vi "Processing.vi"() -> ()   [LabVIEW 2016]
uses:
  Processing/results_data.ctl
  MainFGV/Settings/Advanced/AdvancedConfig.ctl
  Post_processing/GraphMean/data_mean_plot.ctl
  Post_processing/GraphMean/plot_props.ctl
  Post_processing/GraphMean/axis_props.ctl
  <vilib>/Heliosphere Research LLC/Advanced Plotting Toolkit/api_core/NewPlotScales.ctl
  <vilib>/Analysis/NI_AALPro.lvlib
  <vilib>/Heliosphere Research LLC/Advanced Plotting Toolkit/Advanced Plotting Toolkit.lvlib
panel:
  in  "stop":bool
  in  "ranges":T1(array[cluster])=[{"minFreq"=0.0, "maxFreq"=1000.0, "alpha"=20.0}] caption="Ranges de procura de picos" {"alpha" min=0.0 max=100.0 format="%#_6f %"; "maxFreq" format="%#_g Hz"; "minFreq" format="%#_g Hz"}
  in  "log":bool
  in  "alpha":dbl=0.3 caption="Alpha" format="%#_6f"
  in  "maxFreq":dbl=72.0 caption="Frequência máxima" format="%#_g Hz"
  in  "minFreq":dbl=30.0 caption="Frequência mínima" format="%#_g Hz"
  in  "lowPass":dbl=1000.0 caption="Passa baixa" format="%#_g Hz"
  in  "highPass":dbl=1.0 caption="Passa alta" format="%#_g Hz"
  in  "Filtro":T2(ring)=enum."Passa banda"
  in  "cutoff":dbl=-6.0 caption="Cutoff amplitude [dB]" format="%#_g dB"
  in  "delete":bool
  in  "ok":bool
  in  "validate":bool
  in  "tab":T3(tab)
  out "inert":waveform(dbl)[](graph) caption="Inertância"
  out "hammerSpec":waveform(dbl)(graph) caption="Martelo - Espectro"
  out "acelTime":waveform(dbl)[](graph) caption="Acelerômetros - Sinal no tempo"
  out "hammerTime":waveform(dbl)(graph) caption="Martelo - Sinal no tempo"
  out "meanInert":picture
  out "Frequências":dbl[][](array[numeric])
  out "Picos":cluster{"freqs":dbl[], "Array":dbl[]}[](graph) caption="XY Graph"
  in  "TestDir":path=path "C:/Users/l01481/Desktop/nada" caption="Diretório do ensaio"
  # "Análise modal\n\nAquisição\n\nLink do repositório: https://github.com/LeonardoSirino/ModalAnalysis"
  # "Configurações para\napresentação"
  # "Leonardo Sirino\nSistemas Mecânicos \nT + 55 (41) 3361-6152 | C + 55 (41) 99679-007\nleonardo.sirino@lactec.org.br | www.lactec.org.br"
  # "Configurações para\nprocessamento"
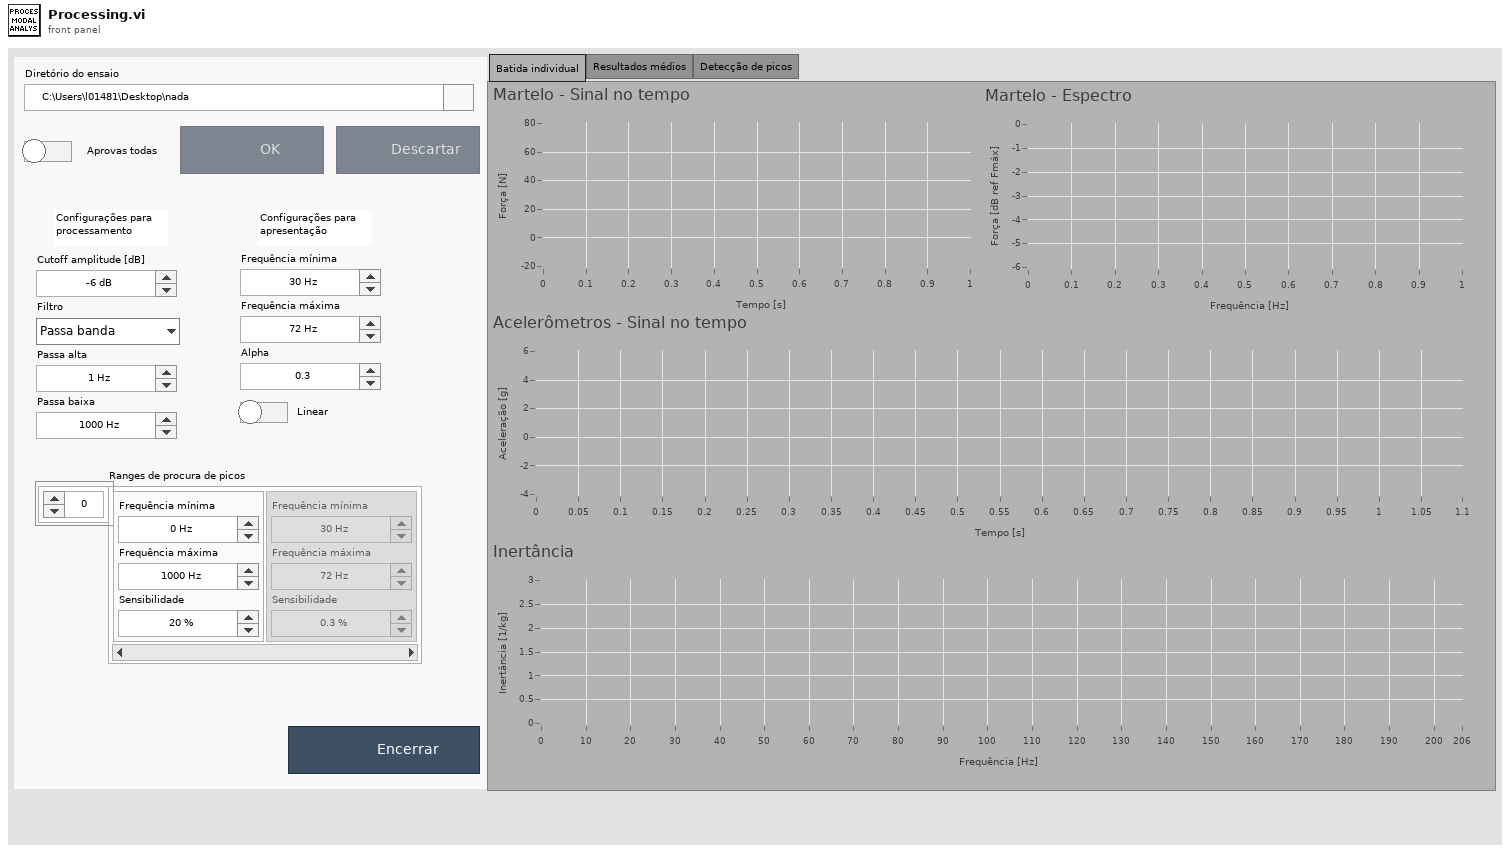
[diagram p1: front panel]
types:
  T1 = cluster{"minFreq":dbl, "maxFreq":dbl, "alpha":dbl}[]
  T2 = enum16{"Desativado", "Passa banda", "Passa alta", "Passa baixa"}
  T3 = enum32{"Batida individual", "Resultados médios", "Detecção de picos"}
  T4 = enum8{"Enabled", "Disabled", "Disabled and Grayed Out"}
  T5 = typedef "AdvancedConfig.ctl" = cluster{"rate":dbl, "duration":dbl, "thr":dbl, "preTrigger":dbl, "cutoff":dbl, "Filtro":enum16{"Desativado", "Passa banda", "Passa alta", "Passa baixa"}, "highPass":dbl, "lowPass":dbl, "updateTime":dbl}
  T6 = typedef "results_data.ctl" = cluster{"config":T5, "hammer":waveform(dbl), "acelerometers":waveform(dbl)[], "hammerIndex":i32}
  T7 = cluster{"seconds since 1Jan1904":timestamp, "data_out":T6}
  T8 = cluster{"seconds since 1Jan1904":timestamp, "data_out":T6}[]
  T9 = typedef "data_mean_plot.ctl" = cluster{"array":dbl[], "dx":dbl, "x0":dbl}
  T10 = typedef "Advanced Plotting Toolkit.lvlib/NewPlotScales.ctl" = enum16{"Default", "Linear", "Log", "Symlog"}
  T11 = typedef "plot_props.ctl" = cluster{"x_axis":T12, "y_axis":T12, "y multiplier":dbl, "alpha":dbl, "base_tag":string, "itens_base_name":string, "graph_title":string, "plot_names":string[], "plot_all":bool}
  T12 = typedef "axis_props.ctl" = cluster{"min":dbl, "max":dbl, "label":string, "scale":T10}
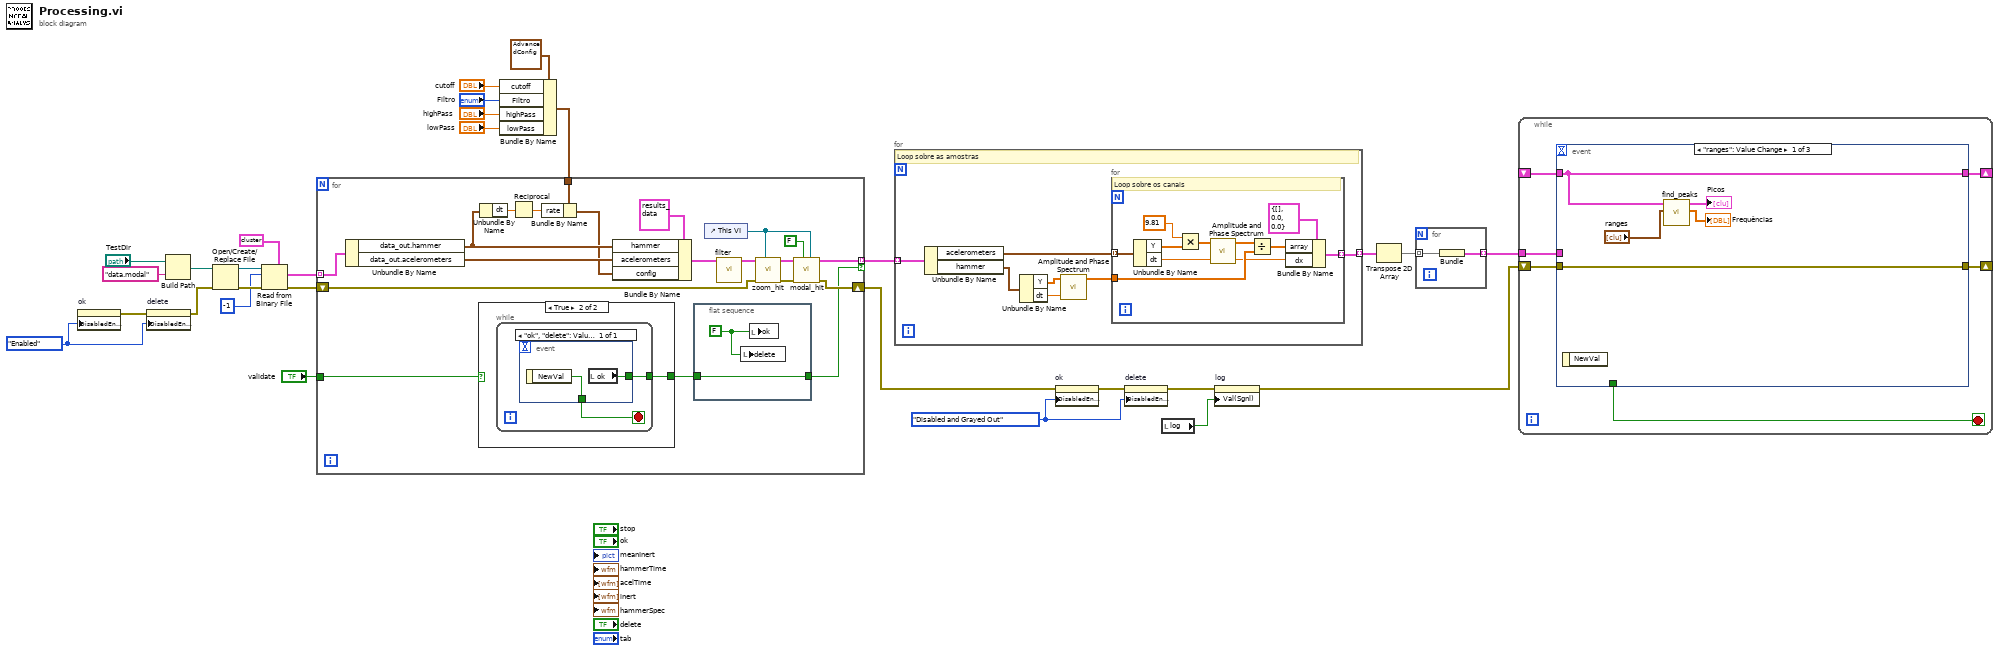
[diagram p0: block diagram]
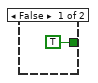
[diagram p2: hidden frame]
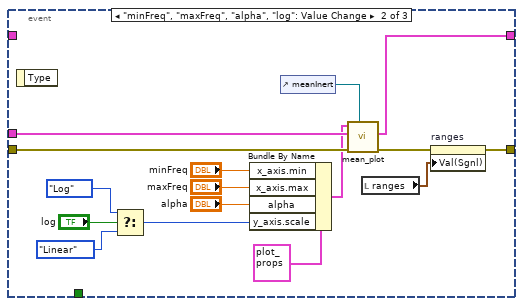
[diagram p3: hidden frame]
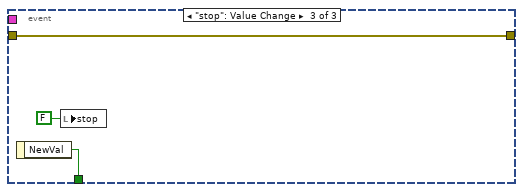
[diagram p4: hidden frame]
diagram:
  w3 = T4."Enabled" ("Disabled")
  w5 = T4."Disabled and Grayed Out" ("Disabled")
  n1 = property on="ok" class="Bool (strict)"("DisabledEnum"=w3) -> (error out=w2:errorcluster)  [unwired: 2 in, 1 out]
  n2 = property on="delete" class="Bool (strict)"(error in=w2, "DisabledEnum"=w3) -> (error out=w1:errorcluster)  [unwired: 1 in, 1 out]
  n3 = Build Path(base path="TestDir", name or relative path="data.modal") -> (appended path=w27:path)
  n4 = Open/Create/Replace File(file path (use dialog)=w27, error in=w1) -> (refnum out=w26:refnum<file>, error out=w24:errorcluster)  [unwired: 4 in, 1 out]
  n5 = Read from Binary File(5:T7 {"seconds since 1Jan1904"=timestamp(0 s since 1904-01-01), "data_out"={"config"={"rate"=0.0, "duration"=0.0, "thr"=0.0, "preTrigger"=0.0, "cutoff"=0.0, "Filtro"=enum."Desativado", "highPass"=0.0, "lowPass"=0.0, "updateTime"=0.0}, "hammer"={"t0"=timestamp(0 s since 1904-01-01), "dt"=1.0, "Y"=[]}, "acelerometers"=[], "hammerIndex"=0}} ("output cluster"), 8:w24, 10:-1 ("count (1)"), 11:w26) -> (0:w15:errorcluster, 2:w22:T8)  [unwired: 2 in, 2 out]
  n6 = Bundle By Name(cluster=T5 {"rate"=1652.0, "duration"=1.0, "thr"=10.0, "preTrigger"=100.0, "cutoff"=-6.0, "Filtro"=enum."Passa banda", "highPass"=1.0, "lowPass"=1000.0, "updateTime"=50.0} ("config"), "cutoff"="cutoff", "Filtro"="Filtro", "highPass"="highPass", "lowPass"="lowPass") -> (w16:T5)
  n7 = for {
    tunnel: w22 -> [w49] mode=indexing
    tunnel: w16 -> [w39]
    shift-right: [w34] -> w7
    shift-left: w15 -> [w35]
    tunnel: [w32] -> w13 mode=indexing if=w31
    tunnel: "validate" -> [w30]
    n8 = Unbundle By Name(w49) -> ("data_out.hammer"=w40:waveform(dbl), "data_out.acelerometers"=w44:waveform(dbl)[])
    n9 = case shown="True" w30 {
      tunnel: [TRUE ("ok") w53] -> w33
      frame False {
      }
      frame True {
        n10 = while {
          tunnel: [w55] -> w53
          stop <- w54 stop-if-true
          n11 = event shown="[0] \"ok\", \"delete\": Value Change" {
            selector: _ -> [_]
            dyn-events: _ -> [_]
            timeout: _ -> [_]
            tunnel: [w56] -> w55
            tunnel: [w57] -> w54
            event "ok", "delete": Value Change {
              n12 = event-data() -> ("NewVal"=w57:bool)  [unwired: 1 in]
              n13 = local read "ok"() -> (w56:bool)
            }
          }
        }
      }
    }
    n14 = Unbundle By Name(w40) -> ("dt"=w38:dbl)
    n15 = Reciprocal(x=w38) -> (1/x=w37:dbl)
    n16 = Bundle By Name(cluster=w39, "rate"=w37) -> (w36:T5)
    n17 = Bundle By Name(cluster=T6 {"config"={"rate"=0.0, "duration"=0.0, "thr"=0.0, "preTrigger"=0.0, "cutoff"=0.0, "Filtro"=enum."Desativado", "highPass"=0.0, "lowPass"=0.0, "updateTime"=0.0}, "hammer"={"t0"=timestamp(0 s since 1904-01-01), "dt"=1.0, "Y"=[]}, "acelerometers"=[], "hammerIndex"=0} ("data_in"), "hammer"=w40, "acelerometers"=w44, "config"=w36) -> (w43:T6)
    n18 = flat-sequence {
      tunnel: w33 -> [w51]
      tunnel: [w51] -> w31
      frame #0 {
        w50 = FALSE ("ok")
        n19 = local write "delete"(w50) -> ()
        n20 = local write "ok"(w50) -> ()
      }
    }
    n21 = control-ref of="This VI"() -> (w42:refnum<vi>)
    n22 = call "filter.vi"("data_in"=w43) -> ("data_out"=w46:T6)  [unwired: 10 in]
    n23 = call "zoom_hit.vi"("refVI"=w42, "error in"=w35, "data_in"=w46) -> ("error out"=w47:errorcluster, "data_out"=w48:T6)  [unwired: 7 in]
    n24 = call "modal_hit.vi"("refVI"=w42, "acquisition"=FALSE, "error in"=w47, "data_in"=w48) -> ("error out"=w34:errorcluster, "data_out"=w32:T6)  [unwired: 6 in]
  }
  n25 = for {
    tunnel: w13 -> [w64] mode=indexing
    tunnel: [w58] -> w12 mode=indexing
    # "Loop sobre as amostras"
    n26 = Unbundle By Name(w64) -> ("acelerometers"=w63:waveform(dbl)[], "hammer"=w60:waveform(dbl))
    n27 = Unbundle By Name(w60) -> ("Y"=w61:dbl[], "dt"=w62:dbl)
    n28 = call <vilib>:"Amplitude and Phase Spectrum.vi"("dt"=w62, "Signal (V)"=w61) -> ("Amp Spectrum Mag (Vrms)"=w59:dbl[])  [unwired: 1 in, 2 out]
    n29 = for {
      tunnel: w63 -> [w75] mode=indexing
      tunnel: w59 -> [w69]
      tunnel: [w65] -> w58 mode=indexing
      # "Loop sobre os canais"
      n30 = Unbundle By Name(w75) -> ("Y"=w74:dbl[], "dt"=w71:dbl)
      n31 = Multiply(x=9.81, y=w74) -> (x*y=w72:dbl[])
      n32 = call <vilib>:"Amplitude and Phase Spectrum.vi"("dt"=w71, "Signal (V)"=w72) -> ("df"=w66:dbl, "Amp Spectrum Mag (Vrms)"=w70:dbl[])  [unwired: 1 in, 1 out]
      n33 = Divide(x=w70, y=w69) -> (x/y=w67:dbl[])
      n34 = Bundle By Name(cluster=T9 {"array"=[], "dx"=0.0, "x0"=0.0} ("data_mean_plot"), "array"=w67, "dx"=w66) -> (w65:T9)
    }
  }
  n35 = property on="ok" class="Bool (strict)"(error in=w7, "DisabledEnum"=w5) -> (error out=w6:errorcluster)  [unwired: 1 in, 1 out]
  n36 = property on="delete" class="Bool (strict)"(error in=w6, "DisabledEnum"=w5) -> (error out=w4:errorcluster)  [unwired: 1 in, 1 out]
  n37 = local read "log"() -> (w10:bool)
  n38 = property on="log" class="Bool (strict)"(error in=w4, "Val(Sgnl)"=w10) -> (error out=w9:errorcluster)  [unwired: 1 in, 1 out]
  n39 = Transpose 2D Array(2D array=w12) -> (transposed array=w11:T9[][])
  n40 = for {
    tunnel: w11 -> [w77] mode=indexing
    tunnel: [w76] -> w8 mode=indexing
    n41 = Bundle(w77) -> (w76:cluster{T9[]})  [unwired: 1 in]
  }
  n42 = while {
    shift-right: [w82] -> _
    shift-left: _ -> [w83]
    tunnel: w8 -> [w81]
    shift-right: [w80] -> _
    shift-left: w9 -> [w79]
    stop <- w78 stop-if-true
    n43 = event shown="[0] \"ranges\": Value Change" {
      selector: _ -> [_ _ _]
      dyn-events: _ -> [_ _ _]
      timeout: _ -> [_ _ _]
      tunnel: w83 -> [w85 _ _]
      tunnel: [w85 w103 _] -> w82
      tunnel: w81 -> [_ w104 _]
      tunnel: [w84 w90 w106] -> w80
      tunnel: w79 -> [w84 w101 w106]
      tunnel: [_ _ w107] -> w78
      event "ranges": Value Change {
        n44 = event-data() -> ()  [unwired: 1 in, 1 out]
        n45 = call "find_peaks.vi"("ranges"="ranges", "data"=w85) -> ("freqs"=→"Frequências":dbl[][], "plots"=→"Picos":cluster{"Array":dbl[], "Array":dbl[]}[])  [unwired: 7 in, 1 out]
      }
      event "minFreq", "maxFreq", "alpha", "log": Value Change {
        n46 = event-data() -> ()  [unwired: 1 in, 1 out]
        n47 = Select(t=NewPlotScales."Log" ("y_axis.scale"), s="log", f=NewPlotScales."Linear" ("y_axis.scale")) -> (s? t:f=w100:T10)
        n48 = Bundle By Name(cluster=T11 {"x_axis"={"min"=30.0, "max"=72.0, "label"="Frequência [Hz]", "scale"=enum."Default"}, "y_axis"={"min"=nan, "max"=nan, "label"="Inertância [1/kg]", "scale"=enum."Linear"}, "y multiplier"=1.0, "alpha"=0.5, "base_tag"="", "itens_base_name"="", "graph_title"="Inertância média", "plot_names"=[], "plot_all"=TRUE} ("plot_properties"), "x_axis.min"="minFreq", "x_axis.max"="maxFreq", "alpha"="alpha", "y_axis.scale"=w100) -> (w92:T11)
        n49 = control-ref of="meanInert"() -> (w102:refnum<vi>)
        n50 = call "mean_plot.vi"("ref_picture"=w102, "error in"=w101, "channels"=w104, "plot_properties"=w92) -> ("error out"=w91:errorcluster, "mean_curves"=w103:cluster{"freqs":dbl[], "Array":dbl[]}[])  [unwired: 5 in, 1 out]
        n51 = local read "ranges"() -> (w89:T1)
        n52 = property on="ranges" class="Arr (strict)"(error in=w91, "Val(Sgnl)"=w89) -> (error out=w90:errorcluster)  [unwired: 1 in, 1 out]
      }
      event "stop": Value Change {
        n53 = event-data() -> ("NewVal"=w107:bool)  [unwired: 1 in]
        n54 = local write "stop"(FALSE ("stop")) -> ()
      }
    }
  }
